vi "SndPB - Run.vi"(0 "reference in":refnum<class "GSwFormDSP.lvclass">, 5 "error in (no error)":errorcluster) -> (11 "New Cursor Location":dbl, 13 "Is Playing?":bool, 14 "reference out":refnum<class "GSwFormDSP.lvclass">, 19 "error out":errorcluster)   [LabVIEW 2020, in "GSwFormDSP.lvclass"]
uses:
  GSwFormDSP.lvclass
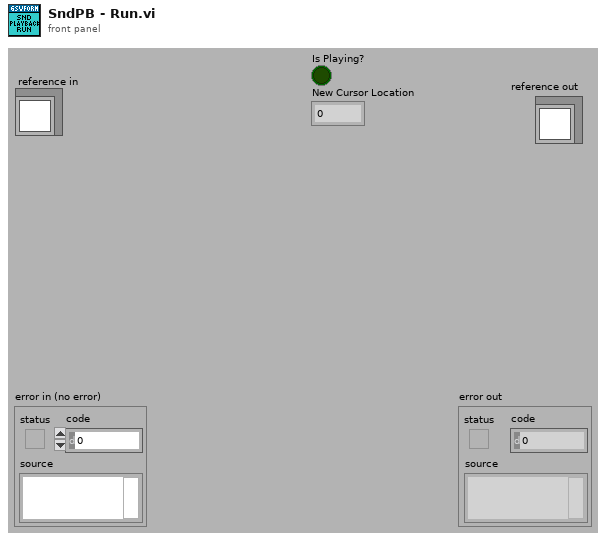
[diagram p1: front panel]
types:
  T1 = typedef "GSwFormDSP.lvclass/Sound Playback.ctl" = cluster{"Timer start (ms)":u32, "task ID":T2, "Cursor Init Location (s)":dbl, "SC Volume":dbl}
  T2 = typedef "Sound Output Task ID.ctl" = u32
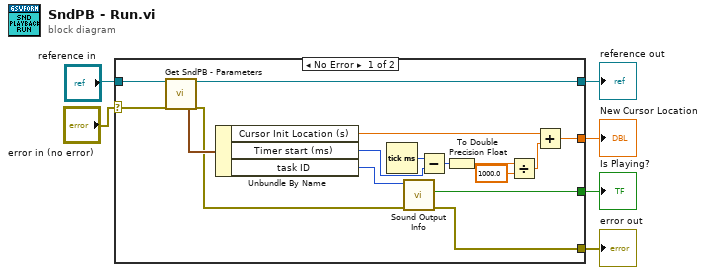
[diagram p0: block diagram]
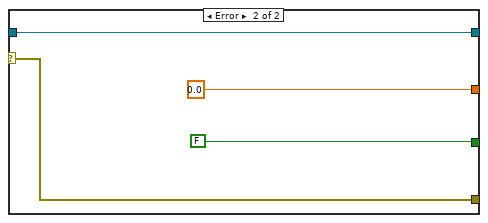
[diagram p2: hidden frame]
diagram:
  n1 = case shown="No Error" "error in (no error)" {
    selector: "error in (no error)" -> [w17 w26]
    tunnel: [w9 w26] -> w5
    tunnel: [w10 w25] -> w3
    tunnel: "reference in" -> [w22 w25]
    tunnel: [w7 FALSE] -> w2
    tunnel: [w8 0.0] -> w1
    frame No Error {
      n2 = call "Get SndPB - Parameters.vi"("reference in"=w22, "error in (no error)"=w17) -> ("Sound Playback"=w21:T1, "reference out"=w10:refnum<class "GSwFormDSP.lvclass">, "error out"=w16:errorcluster)  [unwired: 15 in]
      n3 = Unbundle By Name(w21) -> ("Cursor Init Location (s)"=w20:dbl, "Timer start (ms)"=w19:u32, "task ID"=w18:T2)
      n4 = Tick Count (ms)() -> (millisecond timer value=w14:u32)
      n5 = call <vilib>:"Sound Output Info.vi"("error in (no error)"=w16, "task ID"=w18) -> ("error out"=w9:errorcluster, "is playing?"=w7:bool)  [unwired: 6 in, 2 out]
      n6 = Subtract(x=w14, y=w19) -> (x-y=w15:u32)
      n7 = To Double Precision Float(number=w15) -> (double precision float=w13:dbl)
      n8 = Divide(x=w13, y=1000.0) -> (x/y=w11:dbl)
      n9 = Add(x=w20, y=w11) -> (x+y=w8:dbl)
    }
    frame Error {
    }
  }
  "error out" <- w5
  "reference out" <- w3
  "Is Playing?" <- w2
  "New Cursor Location" <- w1
